vi "Excel Easy Title.vi"(0 "report in":refnum<class "NI_report.lvclass">, 1 "font settings source":u16(ring) items=["VI Inputs", "Font Dialog Box"], 5 "title":string, 7 "start (0, 0)":cluster{"row":i32, "column":i32}, 9 "font":T1={"font name"="", "font size"=18.0, "bold"=1, "italic"=0, "underline"=0, "strike through"=0, "font color"=16777216} {"font size" format="%0.2f"; "strike through" items=["Unchanged", "Yes", "No"]; "underline" items=["Unchanged", "Yes", "No"]; "italic" items=["Unchanged", "Yes", "No"]; "bold" items=["Unchanged", "Yes", "No"]}, 11 "error in (no error)":errorcluster, 12 "name (\"\")":string) -> (4 "report out":refnum<class "NI_report.lvclass">, 6 "font out":T1={"font name"="", "font size"=10.0, "bold"=0, "italic"=0, "underline"=0, "strike through"=0, "font color"=16777216} {"font size" format="%0.2f"; "strike through" items=["Unchanged", "Yes", "No"]; "underline" items=["Unchanged", "Yes", "No"]; "italic" items=["Unchanged", "Yes", "No"]; "bold" items=["Unchanged", "Yes", "No"]}, 15 "error out":errorcluster)   [LabVIEW 2016, in "NI_ReportGenerationToolkit.lvlib"]
doc: "Adds a title to a Microsoft Excel report."
uses:
  <vilib>/addons/_office/NI_ReportGenerationToolkit.lvlib
  <vilib>/Utility/NIReport.llb/NI_report.lvclass
  <vilib>/addons/_office/_exclsub.llb/font.ctl
  <vilib>/Utility/NIReport.llb/Append Report Text (str wrap).vi
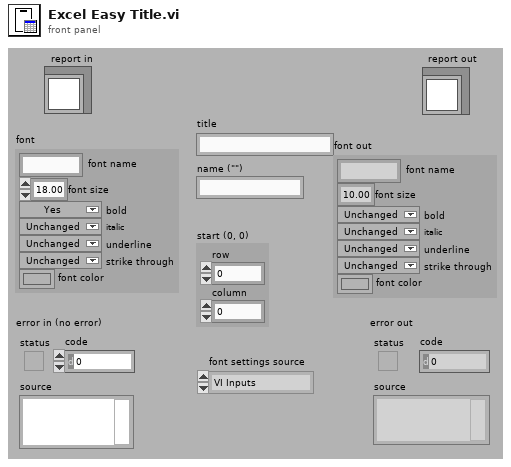
[diagram p1: front panel]
types:
  T1 = typedef "NI_ReportGenerationToolkit.lvlib/font.ctl" = cluster{"font name":string, "font size":dbl, "bold":u16, "italic":u16, "underline":u16, "strike through":u16, "font color":u32}
  T2 = cluster{"position (excel)":cluster{"row":i32, "column":i32}, "name (excel)":string, "bookmark (word)":string}
  T3 = cluster{"Charset (-1)":i16, "Weight (-1)":i16, "Name":string, "Size":string}
  T4 = cluster{i32, i32, i32, i32, "charset":i16, "weight":i16, "name":string, "size":string, "text color":u32}
  T5 = cluster{"italic":u16, "strike through":u16, "underline":u16, "bold":u16}
  T6 = typedef "NI_ReportGenerationCore.lvlib/font.ctl" = cluster{"font name":string, "font size":dbl, "bold":u16, "italic":u16, "underline":u16, "strike through":u16, "font color":u32}
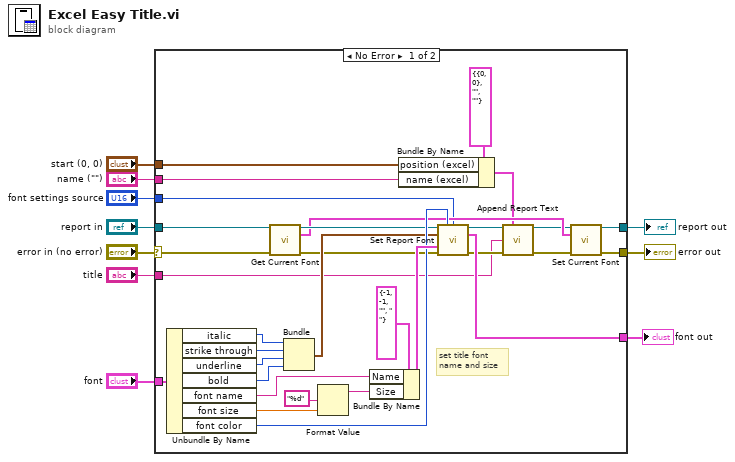
[diagram p0: block diagram]
diagram:
  n1 = case shown="No Error" "error in (no error)" {
    selector: "error in (no error)" -> [w19 w42]
    tunnel: "font" -> [w33 _]
    tunnel: "start (0, 0)" -> [w29 _]
    tunnel: "name (\"\")" -> [w28 _]
    tunnel: "report in" -> [w26 w43]
    tunnel: [w24 w42] -> w6
    tunnel: [w23 w43] -> w5
    tunnel: "font settings source" -> [w21 _]
    tunnel: [w20 _] -> w3
    tunnel: "title" -> [w12 _]
    frame No Error {
      # "set title font\nname and size"
      n2 = Unbundle By Name(w33) -> ("italic"=w34:u16, "strike through"=w37:u16, "underline"=w36:u16, "bold"=w35:u16, "font name"=w18:string, "font size"=w39:dbl, "font color"=w32:u32)
      n3 = call <vilib>:"Get Current Font.vi"("report in"=w26, "error in (no error)"=w19) -> ("report.lvclass"=w25:refnum<class "NI_report.lvclass">, "font"=w22:T4, "error out"=w27:errorcluster)  [unwired: 11 out]
      n4 = Bundle("italic"=w34, "strike through"=w37, "underline"=w36, "bold"=w35) -> (w31:T5)  [unwired: 1 out]
      n5 = Format Value(format string="%d", value (0)=w39) -> (output string=w17:string)  [unwired: 1 out]
      n6 = Bundle By Name(cluster=T3 {"Charset (-1)"=-1, "Weight (-1)"=-1, "Name"="", "Size"=" "} ("font settings"), "Name"=w18, "Size"=w17) -> (w41:T3)
      n7 = Bundle By Name(cluster=T2 {"position (excel)"={"row"=0, "column"=0}, "name (excel)"="", "bookmark (word)"=""} ("MS Office parameters"), "position (excel)"=w29, "name (excel)"=w28) -> (w15:T2)
      n8 = call-dynamic "Set Report Font.vi"("report in"=w25, "text color (unchanged)"=w32, "font settings source (VI Inputs)"=w21, "text options"=w31, "font settings"=w41, "error in (no error)"=w27) -> ("report out"=w11:refnum<class "NI_report.lvclass">, "font out"=w20:T6, "error out"=w14:errorcluster)  [unwired: 7 in]
      n9 = call-poly <vilib>:"Append Report Text.vi"("report in"=w11, "MS Office parameters"=w15, "text"=w12, "error in (no error)"=w14) -> ("report out"=w16:refnum<class "NI_report.lvclass">, "error out"=w13:errorcluster)  [unwired: 2 in, 8 out]
      n10 = call <vilib>:"Set Current Font.vi"("report in"=w16, "font"=w22, "error in (no error)"=w13) -> ("report out"=w23:refnum<class "NI_report.lvclass">, "error out"=w24:errorcluster)  [unwired: 11 out]
    }
    frame Error {
    }
  }
  "report out" <- w5
  "error out" <- w6
  "font out" <- w3
